vi "Get Configuration.vi"(8 "error in (no error)":errorcluster, 11 "Device in":refnum<class "Device.lvclass">) -> (0 "error out":errorcluster, 2 "Configuration":T1, 3 "Device out":refnum<class "Device.lvclass">)   [LabVIEW 2014, in "Device.lvclass"]
uses:
  Device.lvclass
  Device.lvclass/Device.ctl
  Device Configuration/Device Configuration.lvclass/Device Configuration.ctl
  <vilib>/NI/Configuration Framework/serializable configuration/read metadata property.vi
  <vilib>/NI/Configuration Framework/serializable configuration/NISE_CEF_serializable configuration.lvclass
  Device Configuration/Device Configuration.lvclass
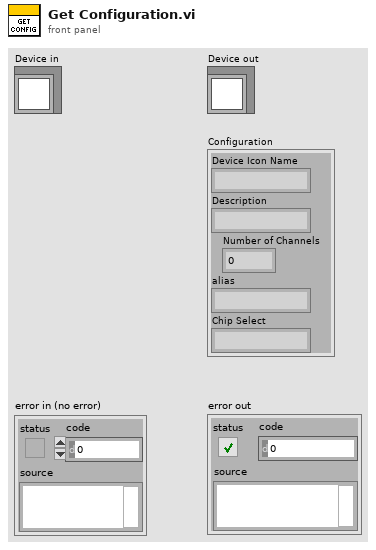
[diagram p1: front panel]
types:
  T1 = cluster{"Device Icon Name":string, "Description":string, "Number of Channels":u32, "alias":string, "Chip Select":string}
  T2 = cluster{"Device Icon Name":string, "Description":string, "Number of Channels":u32, "alias":string, "CS":string}
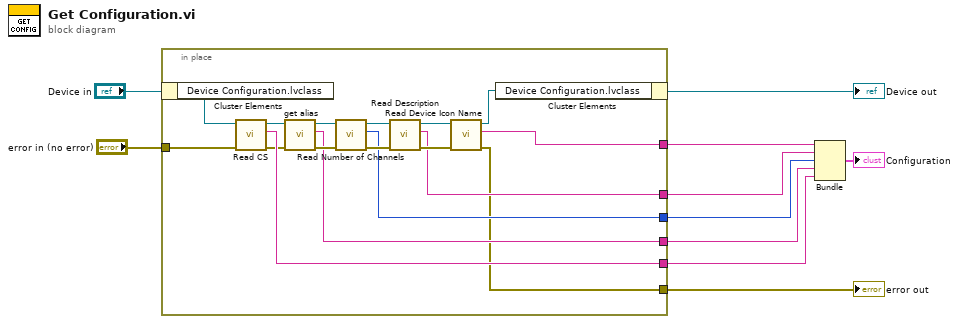
[diagram p0: block diagram]
diagram:
  n1 = in-place {
    in-place-border: [w11] -> w6
    in-place-border: [w18] -> w5
    in-place-border: [w17] -> w4
    in-place-border: [w16] -> w3
    in-place-border: [w15] -> w2
    in-place-border: [w13] -> w8
    in-place-border: "error in (no error)" -> [w12]
    n2 = in-place-cluster #1("Device in") -> ("Device Configuration.lvclass"=w27:refnum<class "Device Configuration.lvclass">)
    n3 = call "Read CS.vi"("error in (no error)"=w12, "Device Configuration in"=w27) -> ("error out"=w14:errorcluster, "CS"=w15:string, "Device Configuration out"=w26:refnum<class "Device Configuration.lvclass">)  [unwired: 7 in]
    n4 = call <vilib>:"get alias.vi"("error in"=w14, "configuration in"=w26) -> ("error out"=w21:errorcluster, "alias"=w16:string, "configuration out"=w25:refnum<class "Device Configuration.lvclass">)  [unwired: 7 in]
    n5 = call "Read Number of Channels.vi"("error in (no error)"=w21, "Device Configuration in"=w25) -> ("error out"=w20:errorcluster, "Number of Channels"=w17:u32, "Device Configuration out"=w24:refnum<class "Device Configuration.lvclass">)  [unwired: 7 in]
    n6 = call "Read Description.vi"("error in (no error)"=w20, "Device Configuration in"=w24) -> ("error out"=w19:errorcluster, "Description"=w18:string, "Device Configuration out"=w23:refnum<class "Device Configuration.lvclass">)  [unwired: 7 in]
    n7 = call "Read Device Icon Name.vi"("error in (no error)"=w19, "Device Configuration in"=w23) -> ("error out"=w13:errorcluster, "Device Icon Name"=w11:string, "Device Configuration out"=w22:refnum<class "Device Configuration.lvclass">)  [unwired: 7 in]
    n8 = in-place-cluster #1("Device Configuration.lvclass"=w22) -> (→"Device out":refnum<class "Device.lvclass">)
  }
  "error out" <- w8
  n9 = Bundle("Device Icon Name"=w6, "Description"=w5, "Number of Channels"=w4, "alias"=w3, "CS"=w2) -> (→"Configuration":T2)  [unwired: 1 in]
